vi "Get topic.vi"(11 "IUnsubscribe in":refnum<class "IUnsubscribe.lvclass">) -> (2 "Topic URl":string, 3 "IUnsubscribe out":refnum<class "IUnsubscribe.lvclass">)   [LabVIEW 2020, in "wamplv.lvlib" / "IUnsubscribe.lvclass"]
uses:
  IUnsubscribe.lvclass
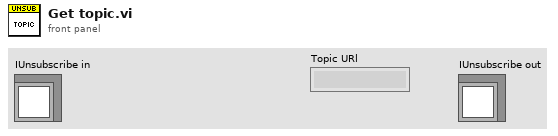
[diagram p1: front panel]
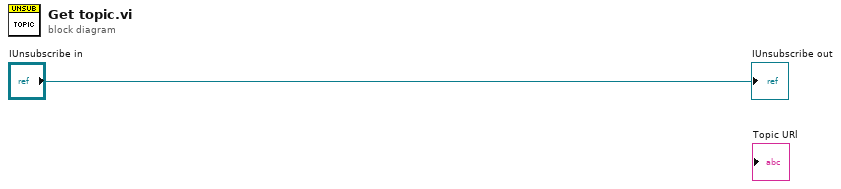
[diagram p0: block diagram]
diagram:
  "IUnsubscribe out" <- "IUnsubscribe in"
